vi "Voltage and Current Ring Chooser.vi"(8 "error in (no error)":errorcluster, 11 "Yokogawa WT2X0 in":refnum<class "Yokogawa WT2X0.lvclass">) -> (0 "error out":errorcluster, 3 "Yokogawa WT2X0 out":refnum<class "Yokogawa WT2X0.lvclass">)   [LabVIEW 2014, in "Generic Power Analyzer.lvlib" / "Yokogawa WT2X0.lvlib" / "Yokogawa WT2X0.lvclass"]
uses:
  Yokogawa WT2X0.lvclass
panel:
  in  "A Range (12: 20A)":u16(ring)=12 items=["Auto", "5mA", "10mA", "20mA", "50mA", "100mA", "200mA", "0.5A", "1A", "2A", "5A", "10A", "20A", "50mV", "100mV", "200mV", "2.5V", "5V", "10V"]
  in  "V Range (6: 600V)":u16(ring)=6 items=["Auto", "15V", "30V", "60V", "150V", "300V", "600V"]
  in  "Wiring (1: 1P3W)":u16(ring)=1 items=["", "1P3W", "3P3W", "3P4W", "3V3A"]
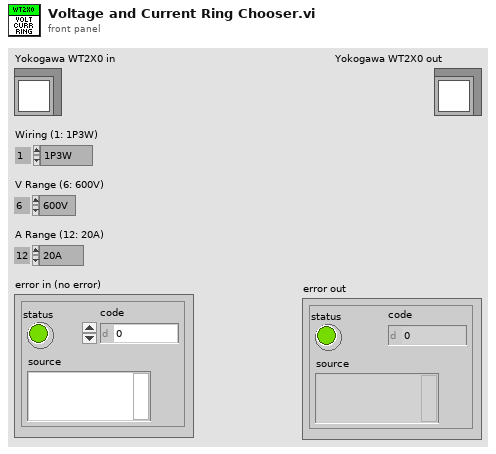
[diagram p1: front panel]
types:
  T1 = typedef "LVStringsAndValuesArrayTypeDef_U16.ctl" = cluster{"String":string, "Value":u16}[]
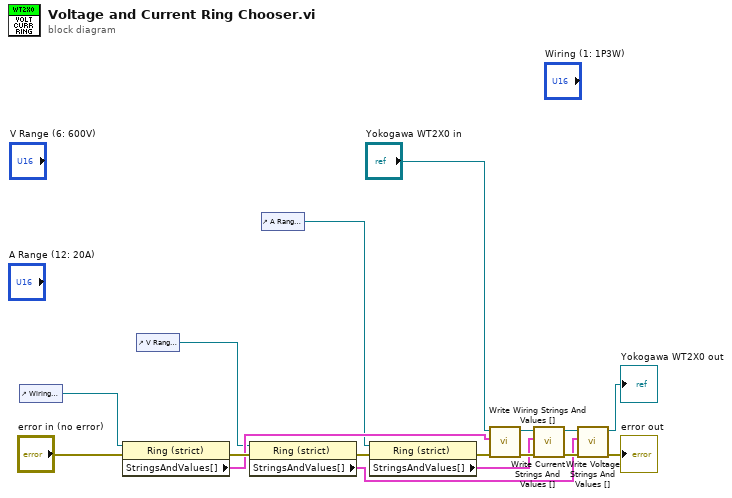
[diagram p0: block diagram]
diagram:
  n1 = control-ref of="Wiring (1: 1P3W)"() -> (w3:refnum<vi>)
  n2 = property class="Ring (strict)"(reference=w3, error in="error in (no error)") -> (error out=w13:errorcluster, "StringsAndValues[]"=w10:T1)  [unwired: 1 out]
  n3 = control-ref of="V Range (6: 600V)"() -> (w2:refnum<vi>)
  n4 = property class="Ring (strict)"(reference=w2, error in=w13) -> (error out=w12:errorcluster, "StringsAndValues[]"=w9:T1)  [unwired: 1 out]
  n5 = control-ref of="A Range (12: 20A)"() -> (w1:refnum<vi>)
  n6 = property class="Ring (strict)"(reference=w1, error in=w12) -> (error out=w11:errorcluster, "StringsAndValues[]"=w8:T1)  [unwired: 1 out]
  n7 = call-dynamic "Write Wiring Strings And Values [].vi"("error in (no error)"=w11, "Strings And Values []"=w10, "Generic Power Analyzer in"="Yokogawa WT2X0 in") -> ("error out"=w15:errorcluster, "Generic Power Analyzer out"=w17:refnum<class "Yokogawa WT2X0.lvclass">)  [unwired: 7 in]
  n8 = call-dynamic "Write Current Strings And Values [].vi"("error in (no error)"=w15, "Strings And Values []"=w8, "Generic Power Analyzer in"=w17) -> ("error out"=w14:errorcluster, "Generic Power Analyzer out"=w16:refnum<class "Yokogawa WT2X0.lvclass">)  [unwired: 7 in]
  n9 = call-dynamic "Write Voltage Strings And Values [].vi"("error in (no error)"=w14, "Strings And Values []"=w9, "Generic Power Analyzer in"=w16) -> ("error out"=→"error out":errorcluster, "Generic Power Analyzer out"=→"Yokogawa WT2X0 out":refnum<class "Yokogawa WT2X0.lvclass">)  [unwired: 7 in]
